vi "Untitled 2.vi"() -> ()   [LabVIEW 2016]
panel:
  in  "Нажмите кнопку":bool
  in  "Какой символ удвоить?":string
  in  "Введите строку":string
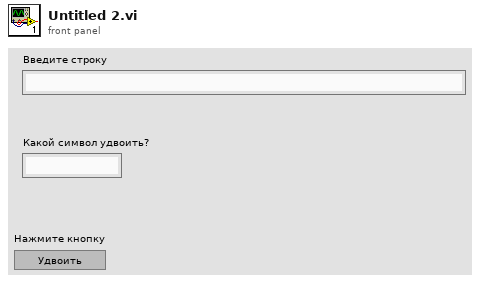
[diagram p1: front panel]
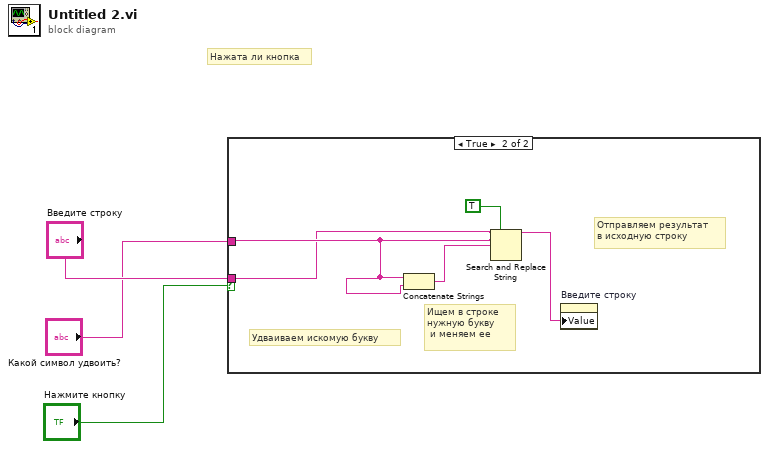
[diagram p0: block diagram]
diagram:
  # "Нажата ли кнопка"
  n1 = case shown="True" "Нажмите кнопку" {
    tunnel: "Введите строку" -> [_ w4]
    tunnel: "Какой символ удвоить?" -> [_ w5]
    frame False {
    }
    frame True {
      # "Отправляем результат \nв исходную строку"
      # "Ищем в строке \nнужную букву\n и меняем ее"
      # "Удваиваем искомую букву"
      n2 = Concatenate Strings(w5, w5) -> (w8:string)
      n3 = Search and Replace String(replace all?=TRUE ("replace all? (F)"), input string=w4, search string=w5, replace string=w8) -> (result string=w6:string)  [unwired: 4 in, 3 out]
      n4 = property on="Введите строку" class="Str"("Value"=w6) -> ()  [unwired: 2 in, 2 out]
    }
  }
